vi "stop.vi"(8 "error in (no error)":errorcluster, 11 "ScanHeadMH100729FPGA in":refnum<class "ScanHeadMH100729FPGA.lvclass">) -> (0 "error out":errorcluster, 3 "ScanHeadMH100729FPGA out":refnum<class "ScanHeadMH100729FPGA.lvclass">)   [LabVIEW 2010, in "ScanHeadMH100729FPGA.lvclass"]
uses:
  ScanHeadMH100729FPGA.lvclass
  Trajectory/GenericTrajectory/GenericTrajectory/GenericTrajectory.lvclass
  Trajectory/TrajectoryMG100122GenericFPGA/TrajectoryMG100122GenericFPGA/TrajectoryMG100122GenericFPGA.lvclass
  common/classes/ErrorController/ErrorController/class_data.vi
  common/classes/ErrorController/ErrorController/ErrorController.lvclass
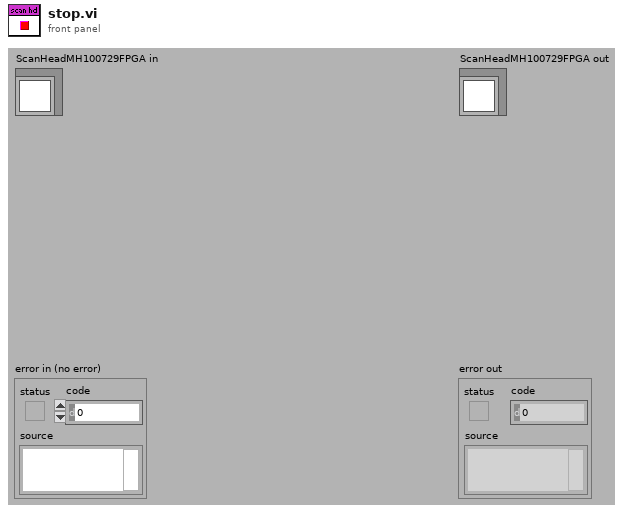
[diagram p1: front panel]
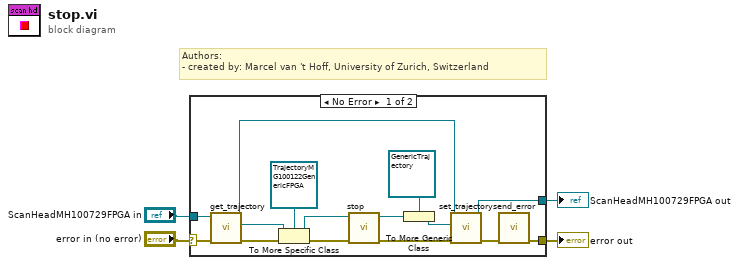
[diagram p0: block diagram]
diagram:
  # "Authors: \n- created by: Marcel van 't Hoff, University of Zurich, Switzerland"
  n1 = case shown="No Error" "error in (no error)" {
    selector: "error in (no error)" -> [w6 w21]
    tunnel: [w7 w21] -> w1
    tunnel: [w15 w20] -> w2
    tunnel: "ScanHeadMH100729FPGA in" -> [w5 w20]
    frame No Error {
      n2 = call-dynamic "get_trajectory.vi"("error in (no error)"=w6, "GenericScanHead.lvclass in"=w5) -> ("error out"=w19:errorcluster, "trajectory"=w9:refnum<class "GenericTrajectory.lvclass">, "GenericScanHead.lvclass out"=w14:refnum<class "ScanHeadMH100729FPGA.lvclass">)  [unwired: 7 in]
      n3 = To More Specific Class(target class=refnum<class "TrajectoryMG100122GenericFPGA.lvclass"> refnum ("TrajectoryMG100122GenericFPGA in"), reference=w9, error in=w19) -> (specific class reference=w11:refnum<class "TrajectoryMG100122GenericFPGA.lvclass">, error out=w13:errorcluster)
      n4 = call-dynamic "stop.vi"("error in (no error)"=w13, "TrajectoryMG100122GenericFPGA in"=w11) -> ("error out"=w12:errorcluster, "TrajectoryMG100122GenericFPGA out"=w10:refnum<class "TrajectoryMG100122GenericFPGA.lvclass">)  [unwired: 8 in]
      n5 = To More Generic Class(target class=refnum<class "GenericTrajectory.lvclass"> refnum ("GenericTrajectory.lvclass"), reference=w10) -> (generic class reference=w16:refnum<class "GenericTrajectory.lvclass">)
      n6 = call-dynamic "set_trajectory.vi"("error in (no error)"=w12, "trajectory"=w16, "GenericScanHead.lvclass in"=w14) -> ("error out"=w8:errorcluster, "GenericScanHead.lvclass out"=w15:refnum<class "ScanHeadMH100729FPGA.lvclass">)  [unwired: 7 in]
      n7 = call "send_error.vi"("error in (no error)"=w8) -> ("error out"=w7:errorcluster)  [unwired: 10 in]
    }
    frame Error {
    }
  }
  "error out" <- w1
  "ScanHeadMH100729FPGA out" <- w2
